vi "Top Level.vi"() -> ()   [LabVIEW 2021, in "Qs.lvlib"]
uses:
  Qs.lvlib
panel:
  in  "Numeric Control":i32
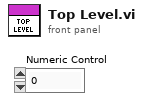
[diagram p1: front panel]
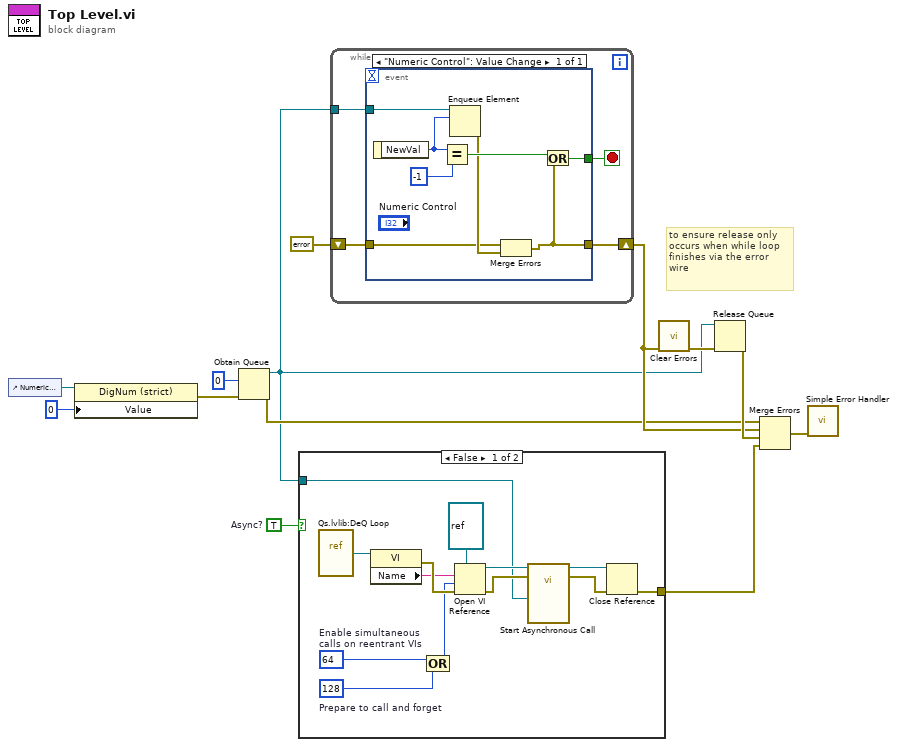
[diagram p0: block diagram]
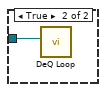
[diagram p2: hidden frame]
diagram:
  w3 = TRUE  # Async?
  # "to ensure release only occurs when while loop finishes via the error wire"
  n1 = control-ref of="Numeric Control"() -> (w13:refnum<vi>)
  n2 = property class="DigNum (strict)"(reference=w13, "Value"=0) -> (error out=w9:errorcluster)  [unwired: 1 in, 1 out]
  n3 = Obtain Queue(element data type=0 ("I32"), error in (no error)=w9) -> (queue out=w2:refnum<queue>, error out=w4:errorcluster)  [unwired: 3 in, 1 out]
  n4 = case shown="False" w3 {
    tunnel: w2 -> [w15 w27]
    tunnel: [w14 _] -> w1
    frame False {
      w21 = 128  # Prepare to call and forget
      w22 = 64  # Enable simultaneous calls on reentrant VIs
      n5 = vi-ref "Qs.lvlib:DeQ Loop.vi"() -> (w25:refnum<vi>)
      n6 = property class="VI"(reference=w25) -> (error out=w24:errorcluster, "Name"=w23:string)  [unwired: 1 in, 1 out]
      n7 = Compound Arithmetic op=OR(w22, w21) -> (w20:i32)
      n8 = Open VI Reference(type specifier VI Refnum (for type only)=refnum<vi> refnum, vi path=w23, options=w20, error in (no error)=w24) -> (vi reference=w18:refnum<vi>, error out=w19:errorcluster)  [unwired: 2 in]
      n9 = call-by-ref "Start Asynchronous Call"(reference=w18, error in=w19, "Queue"=w15) -> (reference out=w16:refnum<vi>, error out=w17:errorcluster)  [unwired: 11 in]
      n10 = Close Reference(reference=w16, error in (no error)=w17) -> (error out=w14:errorcluster)
    }
    frame True {
      n11 = call "DeQ Loop.vi"("Queue"=w27) -> ()  [unwired: 11 in]
    }
  }
  n12 = while {
    shift-right: [w30] -> w5
    shift-left: errorcluster {"status"=FALSE, "code"=0, "source"=""} ("error IO") -> [w29]
    tunnel: w2 -> [w28]
    stop <- w31 stop-if-true
    n13 = event shown="[0] \"Numeric Control\": Value Change" {
      selector: _ -> [_]
      dyn-events: _ -> [_]
      timeout: _ -> [_]
      tunnel: w28 -> [w36]
      tunnel: [w33] -> w31
      tunnel: [w32] -> w30
      tunnel: w29 -> [w34]
      event "Numeric Control": Value Change {
        n14 = event-data() -> ("NewVal"=w37:i32)  [unwired: 1 in]
        n15 = Equal?(x=w37, y=-1) -> (x = y?=w38:bool)
        n16 = Enqueue Element(queue=w36, element=w37) -> (error out=w35:errorcluster)  [unwired: 2 in, 2 out]
        n17 = Merge Errors(w34, w35) -> (w32:errorcluster)
        n18 = Or(x=w38, y=w32) -> (x .or. y?=w33:bool)
      }
    }
  }
  n19 = call <vilib>:"Clear Errors.vi"("error in (no error)"=w5) -> ("error out"=w6:errorcluster)  [unwired: 5 in, 1 out]
  n20 = Release Queue(queue=w2, error in (no error)=w6) -> (error out=w7:errorcluster)  [unwired: 1 in, 2 out]
  n21 = Merge Errors(w4, w5, w7, w1) -> (w10:errorcluster)
  n22 = call <vilib>:"Simple Error Handler.vi"("error in (no error)"=w10) -> ()  [unwired: 4 in, 5 out]
